vi "Process.vi"(8 "error in":errorcluster, 11 "SMO.DynamicLauncher":refnum<class "SMO.DynamicLauncher.lvclass">) -> (0 "error out":errorcluster, 3 "SMO.DynamicLauncher out":refnum<class "SMO.DynamicLauncher.lvclass">)   [LabVIEW 2021, in "SMO.DynamicLauncher.lvclass"]
doc: "---------------------------------------------------------------\nJKI State Machine Objects™\nhttp://jki.net/state-machine-objects/\nCopyright (C) 2005-2015, JKI <info@jki.net>\nALL RIGHTS RESERVED"
uses:
  SMO.DynamicLauncher.lvclass
  SMO.DynamicLauncher.lvclass/SMO.DynamicLauncher.ctl
  src/SMO/SMO.lvclass
  C:/Repositories/SMO/src/SMO/SMO.lvclass
  C:/Repositories/SMO/tests/_test-support-SMOs/SMO.DynamicLauncher/SMO.DynamicLauncher.lvclass
  src/SMO/Typedefs/SMOState --Enum.ctl
panel:
  # "For instructions on how to use the JKI State Machine Objects, examples and video tutorials, visit:\nhttp://jki.net/state-machine-objects/\n\nJKI State Machine Objects™\nhttp://jki.net/state-machine-objects/\nCopyright (C) 2005-2015, JKI <info@jki.net>\nALL RIGHTS RESERVED"
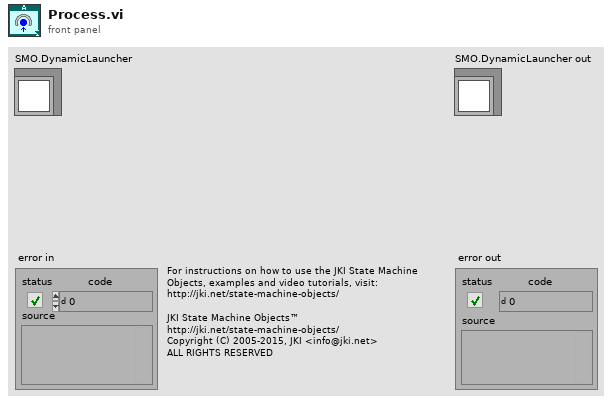
[diagram p1: front panel]
types:
  T1 = enum32{"invalid app kind", "Development System", "Run Time System", "Student Edition", "Embedded LabVIEW", "Evaluation", "Custom"}
  T2 = enum32{"Invalid", "Standard", "Closed", "Hidden", "Minimized", "Maximized"}
  T3 = typedef "smo.lvlib/SMO.lvclass/SMOState --Enum.ctl" = enum16{"unknown", "Created", "Started", "Stopped"}
  T4 = cluster{"Core":cluster{"Current VI Reference":refnum<vi>, "Close Panel on Exit?":bool, "error":errorcluster}, "SelfRef":refnum<class "SMO.DynamicLauncher.lvclass">}
  T5 = cluster{"Current VI Reference":refnum<vi>, "Close Panel on Exit?":bool, "error":errorcluster}
  T6 = typedef "smo.lvlib/SMO.lvclass/Protected Events.ctl" = cluster{"StopProcesses":refnum<user-event>, "AbortProcesses":refnum<user-event>, "Config Changed":refnum<user-event>, "Dependency":refnum<user-event>}
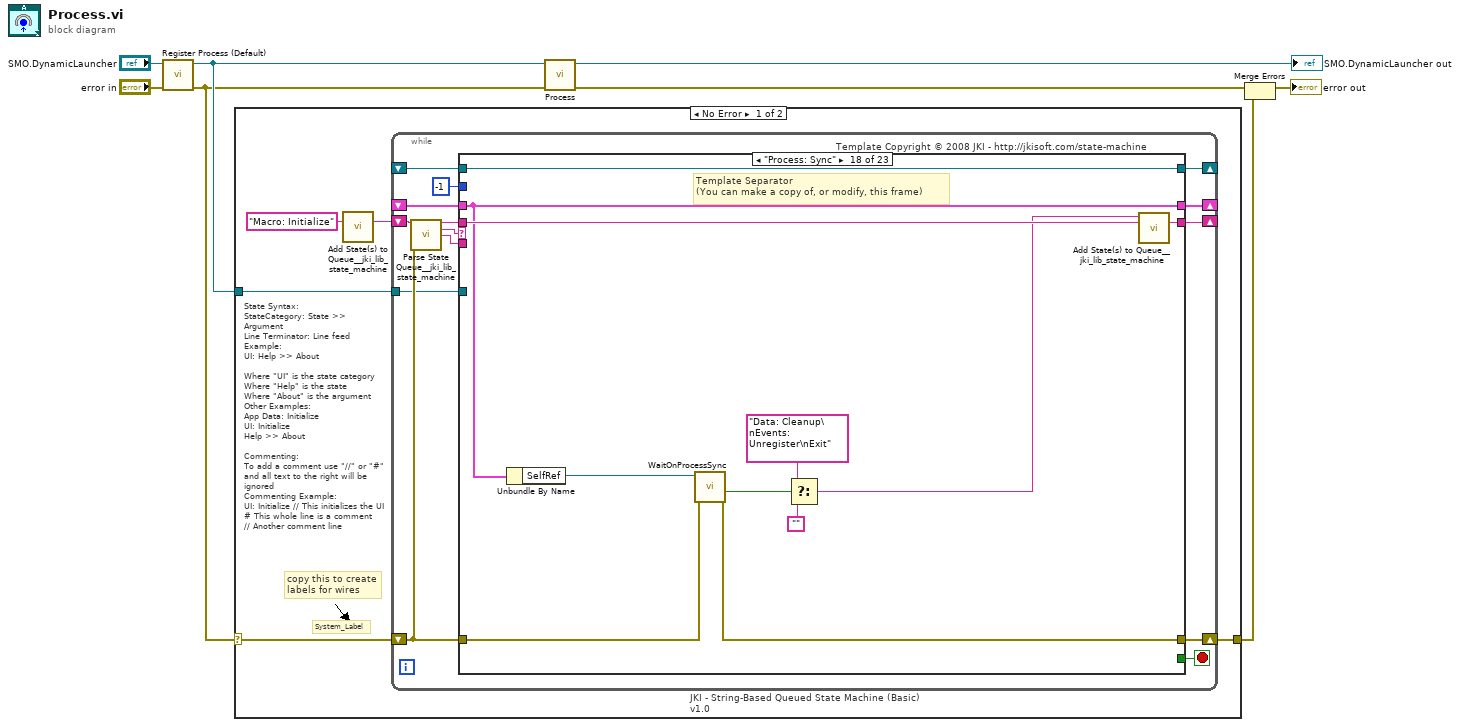
[diagram p0: block diagram]
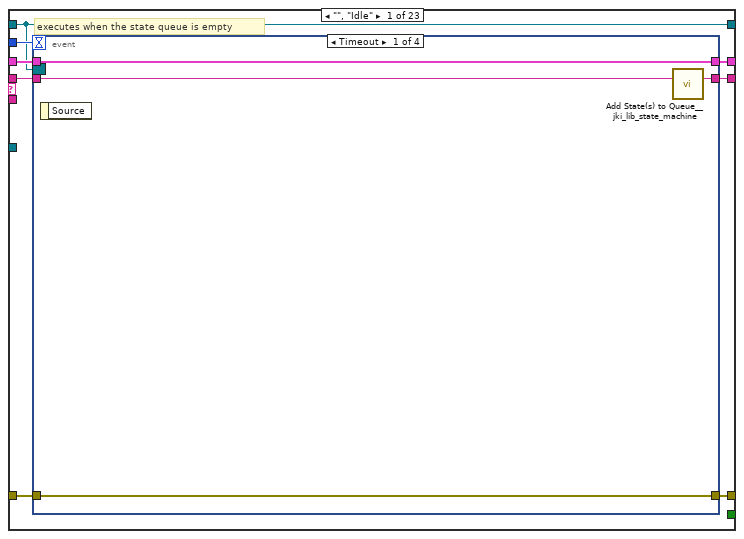
[diagram p2: hidden frame]
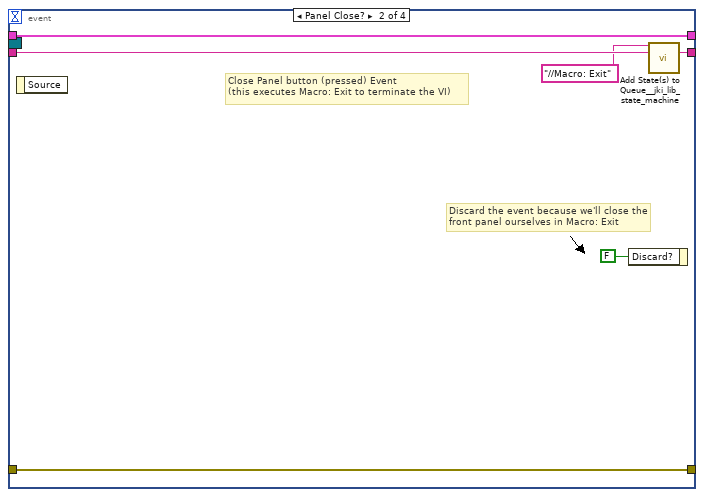
[diagram p3: hidden frame]
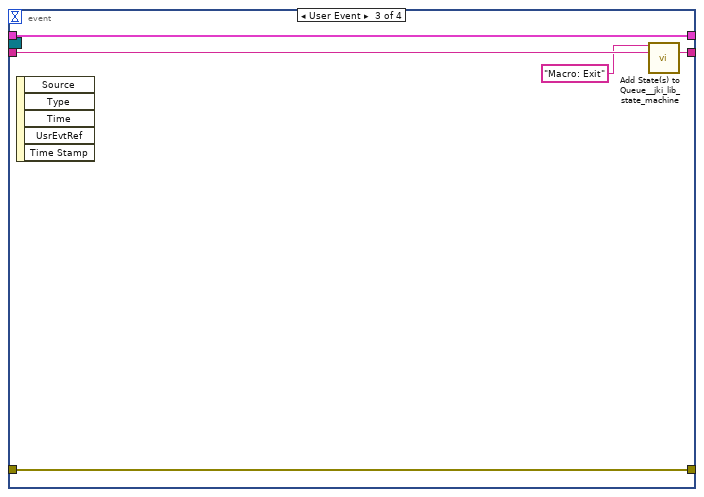
[diagram p4: hidden frame]
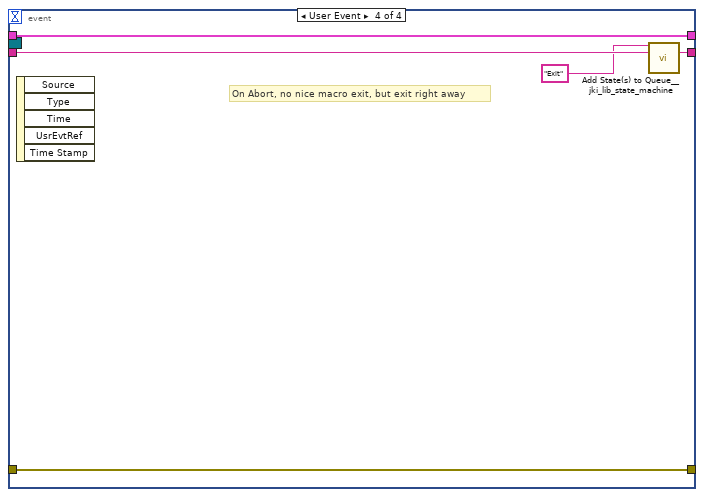
[diagram p5: hidden frame]
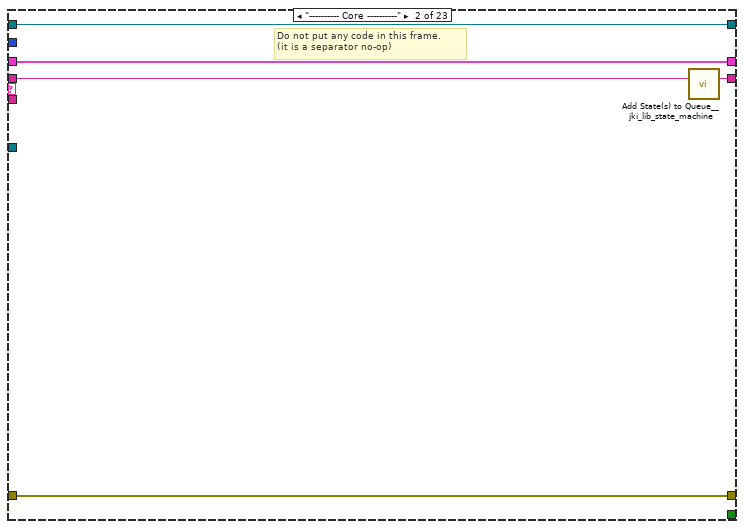
[diagram p6: hidden frame]
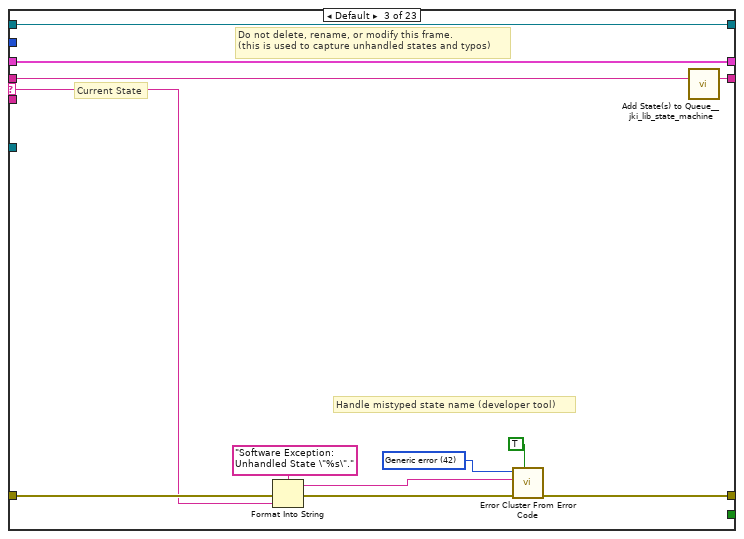
[diagram p7: hidden frame]
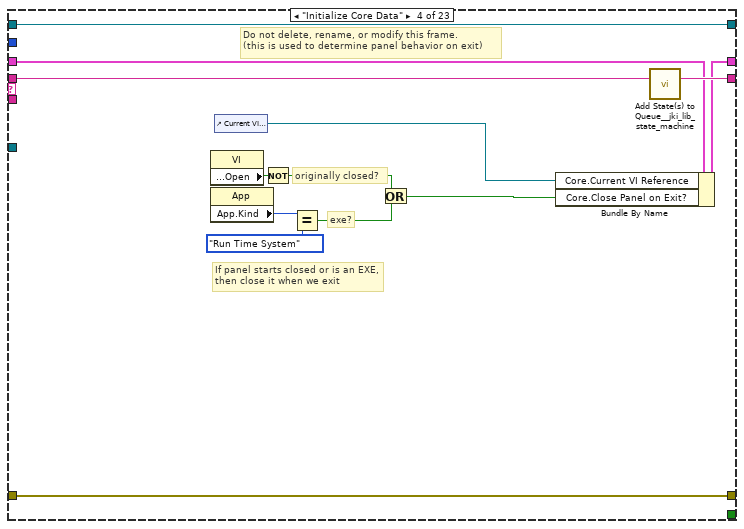
[diagram p8: hidden frame]
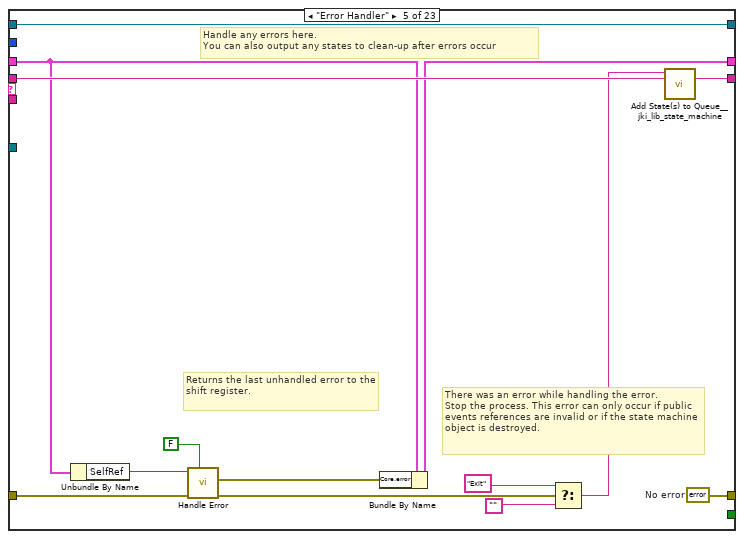
[diagram p9: hidden frame]
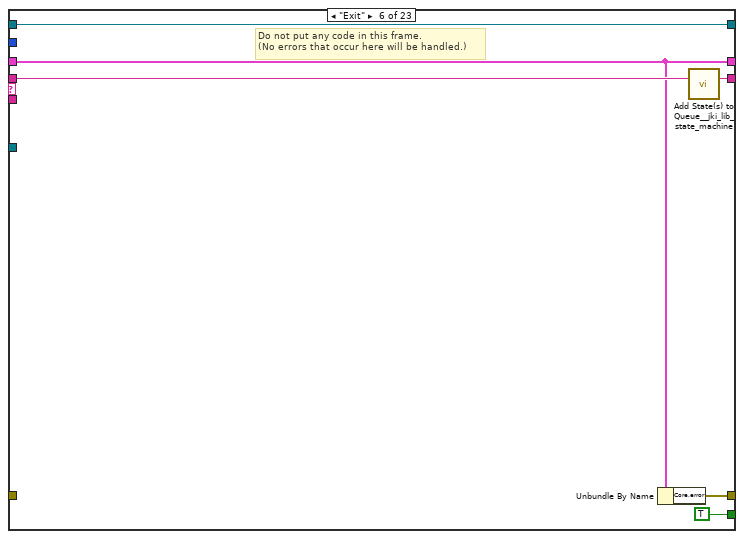
[diagram p10: hidden frame]
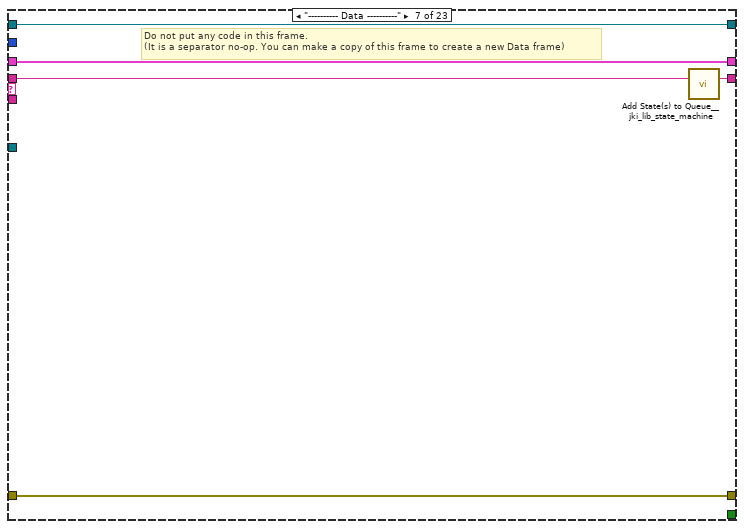
[diagram p11: hidden frame]
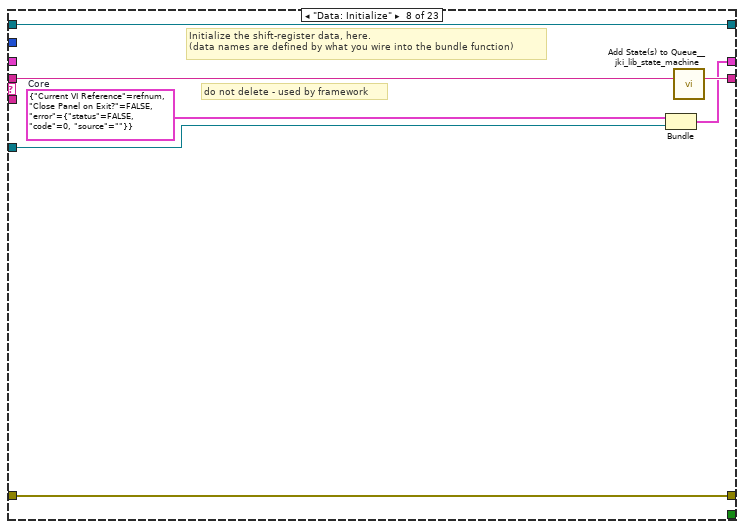
[diagram p12: hidden frame]
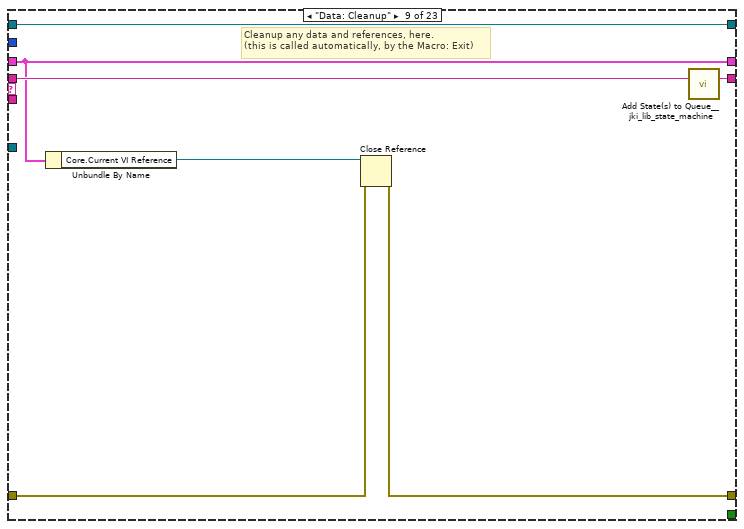
[diagram p13: hidden frame]
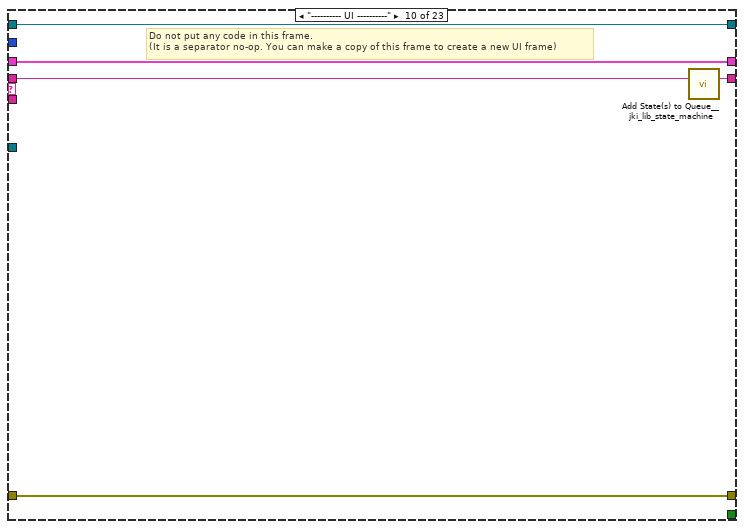
[diagram p14: hidden frame]
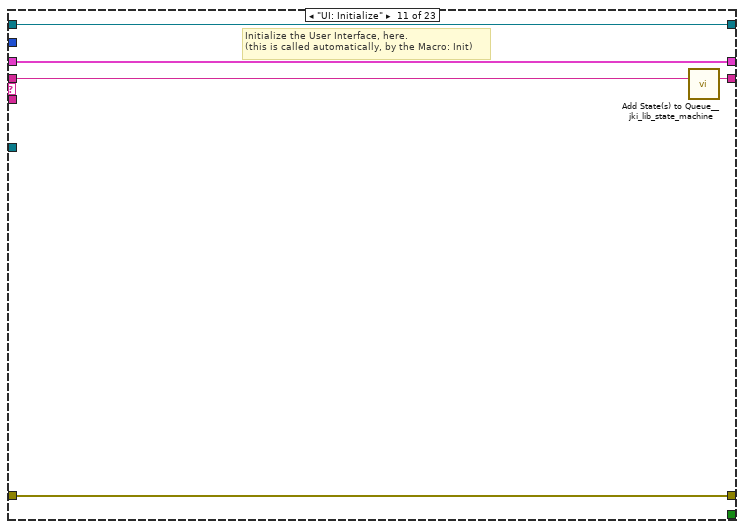
[diagram p15: hidden frame]
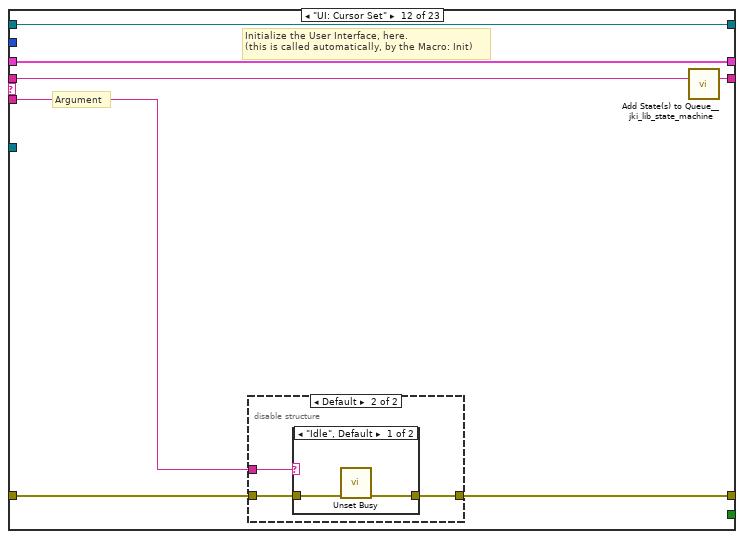
[diagram p16: hidden frame]
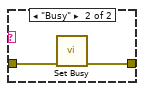
[diagram p18: hidden frame]
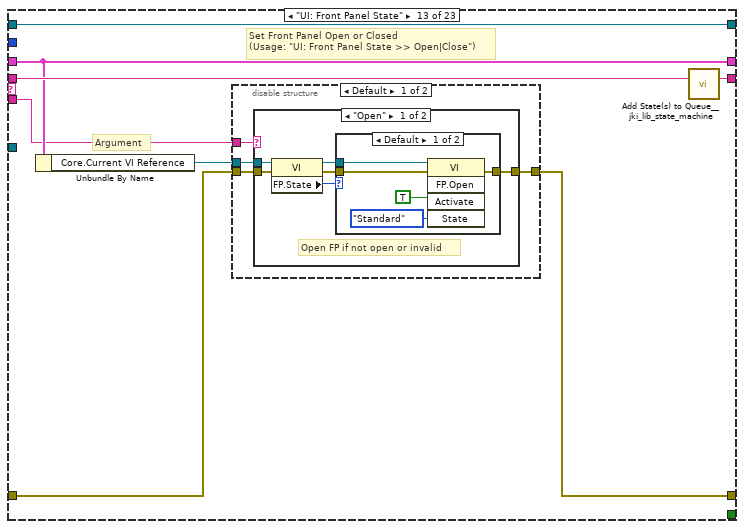
[diagram p19: hidden frame]
diagram:
  n1 = call "Register Process (Default).vi"("error in (no error)"="error in", "SMO"="SMO.DynamicLauncher") -> ("error out"=w1:errorcluster, "SelfRef"=w3:refnum<class "SMO.DynamicLauncher.lvclass">)  [unwired: 8 in]
  n2 = case shown="No Error" w1 {
    selector: w1 -> [w10 w278]
    tunnel: w3 -> [w11 _]
    tunnel: [w9 w278] -> w5
    frame No Error {
      # "State Syntax:\nStateCategory: State >> Argument\nLine Terminator: Line feed\nExample:\nUI: Help >> About\n\nWhere \"UI\" is the state category\nWhere \"Help\" is the state\nWhere \"About\" is the argument\nOther Examples:\nApp Data: Initialize\nUI: Initialize\nHelp >> About\n\nCommenting:\nTo add a comment use \"//\" or \"#\" and all text to the right will be ignored\nCommenting Example:\nUI: Initialize // This initializes the UI\n# This whole line is a comment\n// Another comment line"
      # "copy this to create labels for wires"
      # "System_Label"
      n3 = call <vilib>:"Add State(s) to Queue__jki_lib_state_machine.vi"("State(s) in (\"\")"="Macro: Initialize") -> ("States Out"=w13:string)  [unwired: 14 in]
      n4 = while "JKI - String-Based Queued State Machine (Basic) v1.0" {
        shift-right: [w20] -> _
        shift-left: _ -> [w19]
        shift-right: [w23] -> w9
        shift-left: w10 -> [w17]
        shift-right: [w22] -> _
        shift-left: w13 -> [w24]
        tunnel: w11 -> [w16]
        shift-right: [w15] -> _
        shift-left: _ -> [w14]
        stop <- w21 stop-if-true
        # "Template Copyright © 2008 JKI - http://jkisoft.com/state-machine"
        n5 = call <vilib>:"Parse State Queue__jki_lib_state_machine.vi"("State Queue"=w24, "Error In (no error)"=w17) -> ("Remaining States"=w26:string, "Current State"=w27:string, "Arguments"=w25:string)  [unwired: 11 in]
        n6 = case shown="\"Process: Sync\"" w27 {
          selector: w27 -> [_ _ w62 _ _ _ _ _ _ _ _ _ _ _ _ _ _ _ _ _ _ _ _]
          tunnel: w26 -> [w35 w60 w66 w85 w99 w105 w110 w117 w124 w129 w134 w141 w157 w189 w198 w212 w217 w228 w233 w243 w249 w254 w266]
          tunnel: w25 -> [_ _ _ _ _ _ _ _ _ _ _ w135 w150 _ _ _ _ _ _ _ _ _ _]
          tunnel: w19 -> [w33 w57 w64 w76 w90 w101 w107 _ w119 w126 w132 w139 w155 w186 w194 w203 w214 w225 w230 w241 w247 w252 w263]
          tunnel: [w32 w58 w68 w82 w87 w100 w108 w111 w120 w127 w131 w136 w151 w187 w196 w210 w215 w219 w231 w234 w245 w250 w259] -> w23
          tunnel: w17 -> [w31 w58 w67 w82 w91 _ w108 w111 w121 w127 w131 w137 w152 w187 w196 w210 w215 w220 w231 w235 w245 w250 w260]
          tunnel: [w34 w59 w65 w84 w98 w104 w109 w116 w123 w128 w133 w140 w156 w188 w197 w211 w216 w227 w232 w242 w248 w253 w265] -> w22
          tunnel: [_ _ _ _ _ TRUE _ _ _ _ _ _ _ _ _ _ _ _ _ _ _ _ _] -> w21
          tunnel: [w30 w57 w64 w83 w89 w101 w107 w115 w119 w126 w132 w139 w155 w186 w194 w203 w214 w225 w230 w241 w247 w252 w263] -> w20
          tunnel: -1 -> [w29 _ _ _ _ _ _ _ _ _ _ _ _ _ _ _ _ _ _ _ _ _ _]
          tunnel: w16 -> [_ _ _ _ _ _ _ w112 _ _ _ _ _ _ _ _ _ _ _ _ _ _ _]
          tunnel: [w28 w56 w61 w73 w97 w102 w106 w114 w118 w125 w130 w138 w154 w185 w195 w204 w213 w226 w229 w238 w246 w251 w264] -> w15
          tunnel: w14 -> [w28 w56 w61 w73 w97 w102 w106 w114 w118 w125 w130 w138 w154 w185 w195 w204 w213 w226 w229 _ w246 w251 w264]
          frame "", "Idle" {
            # "executes when the state queue is empty"
            n7 = event shown="[0] Timeout" {
              selector: w28 -> [_ _ _ _]
              dyn-events: _ -> [_ _ _ _]
              timeout: w29 -> [_ _ _ _]
              tunnel: w35 -> [w39 w45 w50 w55]
              tunnel: [w38 w44 w49 w54] -> w34
              tunnel: w33 -> [w36 w42 w47 w52]
              tunnel: [w37 w43 w48 w53] -> w32
              tunnel: w31 -> [w37 w43 w48 w53]
              tunnel: [w36 w42 w47 w52] -> w30
              event Timeout {
                n8 = event-data() -> ()  [unwired: 1 in, 1 out]
                n9 = call <vilib>:"Add State(s) to Queue__jki_lib_state_machine.vi"("State(s) in (\"\")"=w39) -> ("States Out"=w38:string)  [unwired: 14 in]
              }
              event Panel Close? {
                # "Discard the event because we'll close the front panel ourselves in Macro: Exit"
                # "Close Panel button (pressed) Event\n(this executes Macro: Exit to terminate the VI)"
                n10 = event-data() -> ()  [unwired: 1 in, 1 out]
                n11 = event-data("Discard?"=FALSE) -> ()  [unwired: 1 in, 1 out]
                n12 = call <vilib>:"Add State(s) to Queue__jki_lib_state_machine.vi"("State(s) in Front (\"\")"="//Macro: Exit", "State(s) in (\"\")"=w45) -> ("States Out"=w44:string)  [unwired: 13 in]
              }
              event User Event {
                n13 = event-data() -> ()  [unwired: 1 in, 5 out]
                n14 = call <vilib>:"Add State(s) to Queue__jki_lib_state_machine.vi"("State(s) in Front (\"\")"="Macro: Exit", "State(s) in (\"\")"=w50) -> ("States Out"=w49:string)  [unwired: 13 in]
              }
              event User Event {
                # "On Abort, no nice macro exit, but exit right away"
                n15 = event-data() -> ()  [unwired: 1 in, 5 out]
                n16 = call <vilib>:"Add State(s) to Queue__jki_lib_state_machine.vi"("State(s) in Front (\"\")"="Exit", "State(s) in (\"\")"=w55) -> ("States Out"=w54:string)  [unwired: 13 in]
              }
            }
          }
          frame "---------- Core ----------" {
            # "Do not put any code in this frame.\n(it is a separator no-op)"
            n17 = call <vilib>:"Add State(s) to Queue__jki_lib_state_machine.vi"("State(s) in (\"\")"=w60) -> ("States Out"=w59:string)  [unwired: 14 in]
          }
          frame Default {
            w71 = 42 items=["No error", "Argument error", "Memory is full", "Out of zone", "End of file", "File already open", "Generic file I/O error", "File not found", "File permission error", "Disk is full", "Duplicate path", "Too many files open", "System feature not enabled", "Resource file not found", "Cannot add resource", "Resource not found", "Image not found", "Image memory error", "Pen does not exist", "Config type invalid", "Config token not found", "Config parse error", "Config memory error", "Bad external code format", "Bad external code offset", "External code not present", "Null window", "Destroy window error", "Null menu", "Print aborted", "Bad print record", "Print driver error", "Windows error during printing", "Memory error during printing", "Print dialog error", "Generic print error", "Invalid device refnum", "Device not found", "Device parameter error", "Device unit error", "Cannot open device", "Device call aborted", "Generic error", "Cancelled by user", "Object ID too low", "Object ID too high", "Object not in heap", "Unknown heap", "Unknown object (invalid DefProc)", "Unknown object (DefProc not in table)", "Message out of range", "Invalid (null) method", "Unknown message", "Manager call not supported", "Bad address", "Network operation in progress", "Network operation timed out", "Connection is busy", "Network attribute not supported", "Network error", "Address in use", "System out of memory", "Connection aborted", "Connection refused", "Not connected", "Already connected", "Connection closed", "Initialization error (interapplication manager)", "Bad occurrence", "Wait on unbound occurrence handler", "Occurrence queue overflow", "Datalog type conflict", "Unused", "Unrecognized type (interapplication manager)", "Memory corrupt", "Failed to make temporary DLL", "Old CIN version", "Drag socket not found", "Failed to load drop-object", "Failed to register OLE object", "Failed to release OLE object", "Format specifier type mismatch", "Unknown format specifier", "Too few format specifiers", "Too many format specifiers", "Scan failed", "Newer CIN version", "Error converting to variant", "Runtime menu error", "Password tampered", "Variant attribute not found", "Incompatible variant data type", "Event data is not available", "Event Store is not present", "Occurrence is not found", "Event Queue is not created", "Event info is not available", "Refnum passed is NULL", "Error retrieving Class GUID", "Error retrieving CoClass GUID", "Error retrieving TypeLib GUID.", "Bad built application magic bytes.", "Specific driver is different from the specific driver associated with the Logical Name.", "There is no session opened to the class driver.", "Max Error", "MAX - Error with config objects", "MAX - Error loading configuration", "MAX - Group not supported"]
            # "Current State"
            # "Do not delete, rename, or modify this frame.\n(this is used to capture unhandled states and typos)"
            # "Handle mistyped state name (developer tool)"
            n18 = Format Into String(format string="Software Exception: Unhandled State \"%s\"." ("message"), error in=w67, w62) -> (resulting string=w70:string, error out=w69:errorcluster)  [unwired: 1 in]
            n19 = call <vilib>:"Error Cluster From Error Code.vi"("show call chain? (False)"=TRUE, "error in (no error)"=w69, "error message (\"\")"=w70, "error code (0)"=w71) -> ("error out"=w68:errorcluster)  [unwired: 5 in]
            n20 = call <vilib>:"Add State(s) to Queue__jki_lib_state_machine.vi"("State(s) in (\"\")"=w66) -> ("States Out"=w65:string)  [unwired: 14 in]
          }
          frame "Initialize Core Data" {
            # "Do not delete, rename, or modify this frame.\n(this is used to determine panel behavior on exit)"
            # "originally closed?"
            # "exe?"
            # "If panel starts closed or is an EXE, then close it when we exit"
            n21 = property class="VI"() -> ("Front Panel.Open"=w81:bool)  [unwired: 2 in, 2 out]
            n22 = property class="App"() -> ("App.Kind"=w80:T1)  [unwired: 2 in, 2 out]
            n23 = control-ref of="Current VI Reference"() -> (w74:refnum<vi>)
            n24 = Not(x=w81) -> (.not. x?=w78:bool)
            n25 = Equal?(x=w80, y=T1."Run Time System" ("Application:Kind")) -> (x = y?=w77:bool)
            n26 = Or(x=w78, y=w77) -> (x .or. y?=w75:bool)
            n27 = Bundle By Name(cluster=w76, "Core.Current VI Reference"=w74, "Core.Close Panel on Exit?"=w75) -> (w83:T4)
            n28 = call <vilib>:"Add State(s) to Queue__jki_lib_state_machine.vi"("State(s) in (\"\")"=w85) -> ("States Out"=w84:string)  [unwired: 14 in]
          }
          frame "Error Handler" {
            w87 = errorcluster {"status"=FALSE, "code"=0, "source"=""}  # No error
            # "Returns the last unhandled error to the shift register."
            # "There was an error while handling the error.\nStop the process. This error can only occur if public events references are invalid or if the state machine object is destroyed."
            # "Handle any errors here.\nYou can also output any states to clean-up after errors occur"
            n29 = Unbundle By Name(w90) -> ("SelfRef"=w92:refnum<class "SMO.DynamicLauncher.lvclass">)
            n30 = call-dynamic "Handle Error.vi"("Stop on Unhandled Error (T)"=FALSE, "error in"=w91, "SMO"=w92) -> ("handling error"=w94:errorcluster, "Unhandled error"=w93:errorcluster)  [unwired: 6 in, 1 out]
            n31 = Bundle By Name(cluster=w90, "Core.error"=w93) -> (w89:T4)
            n32 = Select(t="Exit", s=w94, f="") -> (s? t:f=w88:string)
            n33 = call <vilib>:"Add State(s) to Queue__jki_lib_state_machine.vi"("State(s) in Front (\"\")"=w88, "State(s) in (\"\")"=w99) -> ("States Out"=w98:string)  [unwired: 13 in]
          }
          frame "Exit" {
            # "Do not put any code in this frame.\n(No errors that occur here will be handled.)"
            n34 = Unbundle By Name(w101) -> ("Core.error"=w100:errorcluster)
            n35 = call <vilib>:"Add State(s) to Queue__jki_lib_state_machine.vi"("State(s) in (\"\")"=w105) -> ("States Out"=w104:string)  [unwired: 14 in]
          }
          frame "---------- Data ----------" {
            # "Do not put any code in this frame.\n(It is a separator no-op. You can make a copy of this frame to create a new Data frame)"
            n36 = call <vilib>:"Add State(s) to Queue__jki_lib_state_machine.vi"("State(s) in (\"\")"=w110) -> ("States Out"=w109:string)  [unwired: 14 in]
          }
          frame "Data: Initialize" {
            w113 = T5 {"Current VI Reference"=refnum, "Close Panel on Exit?"=FALSE, "error"={"status"=FALSE, "code"=0, "source"=""}}  # Core
            # "do not delete - used by framework"
            # "Initialize the shift-register data, here.\n(data names are defined by what you wire into the bundle function)"
            n37 = Bundle("Core"=w113, "SelfRef"=w112) -> (w115:T4)  [unwired: 1 in]
            n38 = call <vilib>:"Add State(s) to Queue__jki_lib_state_machine.vi"("State(s) in (\"\")"=w117) -> ("States Out"=w116:string)  [unwired: 14 in]
          }
          frame "Data: Cleanup" {
            # "Cleanup any data and references, here.\n(this is called automatically, by the Macro: Exit)"
            n39 = Unbundle By Name(w119) -> ("Core.Current VI Reference"=w122:refnum<vi>)
            n40 = Close Reference(reference=w122, error in (no error)=w121) -> (error out=w120:errorcluster)
            n41 = call <vilib>:"Add State(s) to Queue__jki_lib_state_machine.vi"("State(s) in (\"\")"=w124) -> ("States Out"=w123:string)  [unwired: 14 in]
          }
          frame "---------- UI ----------" {
            # "Do not put any code in this frame.\n(It is a separator no-op. You can make a copy of this frame to create a new UI frame)"
            n42 = call <vilib>:"Add State(s) to Queue__jki_lib_state_machine.vi"("State(s) in (\"\")"=w129) -> ("States Out"=w128:string)  [unwired: 14 in]
          }
          frame "UI: Initialize" {
            # "Initialize the User Interface, here.\n(this is called automatically, by the Macro: Init)"
            n43 = call <vilib>:"Add State(s) to Queue__jki_lib_state_machine.vi"("State(s) in (\"\")"=w134) -> ("States Out"=w133:string)  [unwired: 14 in]
          }
          frame "UI: Cursor Set" {
            # "Argument"
            # "Initialize the User Interface, here.\n(this is called automatically, by the Macro: Init)"
            n44 = disable-structure shown="Default" {
              disable-tunnel: w137 -> [w142 w145]
              disable-tunnel: [w142 w144] -> w136
              disable-tunnel: w135 -> [_ w143]
              frame condition #0 {
              }
              frame condition #1 (active) {
                n45 = case shown="\"Idle\", Default" w143 {
                  tunnel: w145 -> [w147 w149]
                  tunnel: [w146 w148] -> w144
                  frame "Idle", Default {
                    n46 = call <vilib>:"Unset Busy.vi"("error in (no error)"=w147) -> ("error out"=w146:errorcluster)  [unwired: 10 in]
                  }
                  frame "Busy" {
                    n47 = call <vilib>:"Set Busy.vi"("error in (no error)"=w149) -> ("error out"=w148:errorcluster)  [unwired: 9 in, 1 out]
                  }
                }
              }
            }
            n48 = call <vilib>:"Add State(s) to Queue__jki_lib_state_machine.vi"("State(s) in (\"\")"=w141) -> ("States Out"=w140:string)  [unwired: 14 in]
          }
          frame "UI: Front Panel State" {
            # "Argument"
            # "Set Front Panel Open or Closed\n(Usage: \"UI: Front Panel State >> Open|Close\")"
            n49 = Unbundle By Name(w155) -> ("Core.Current VI Reference"=w153:refnum<vi>)
            n50 = disable-structure shown="Default" {
              disable-tunnel: w152 -> [w161 w184]
              disable-tunnel: [w160 w184] -> w151
              disable-tunnel: w153 -> [w159 _]
              disable-tunnel: w150 -> [w158 _]
              frame condition #0 (active) {
                n51 = case shown="\"Open\"" w158 {
                  tunnel: w161 -> [w165 w178]
                  tunnel: [w167 w179] -> w160
                  tunnel: w159 -> [w166 w176]
                  frame "Open" {
                    # "Open FP if not open or invalid"
                    n52 = property class="VI"(reference=w166, error in=w165) -> (reference out=w163:refnum<vi>, error out=w164:errorcluster, "FP.State"=w162:T2)
                    n53 = case shown="Default" w162 {
                      tunnel: [w170 w173] -> w167
                      tunnel: w164 -> [w169 w173]
                      tunnel: w163 -> [w168 _]
                      frame Default {
                        n54 = invoke class="VI" method="FP.Open"(reference=w168, error in=w169, "Activate"=TRUE, "State"=T2."Standard") -> (error out=w170:errorcluster)  [unwired: 1 in, 4 out]
                      }
                      frame "Invalid", "Standard" {
                      }
                    }
                  }
                  frame "Close", Default {
                    # "Close FP is not Closed or Invalid"
                    n55 = property class="VI"(reference=w176, error in=w178) -> (reference out=w175:refnum<vi>, error out=w177:errorcluster, "FP.State"=w174:T2)
                    n56 = case shown="Default" w174 {
                      tunnel: [w180 w183] -> w179
                      tunnel: w177 -> [w180 w182]
                      tunnel: w175 -> [_ w181]
                      frame "Invalid", "Closed" {
                      }
                      frame Default {
                        n57 = invoke class="VI" method="FP.Close"(reference=w181, error in=w182) -> (error out=w183:errorcluster)  [unwired: 1 in, 2 out]
                      }
                    }
                  }
                }
              }
              frame condition #1 {
              }
            }
            n58 = call <vilib>:"Add State(s) to Queue__jki_lib_state_machine.vi"("State(s) in (\"\")"=w157) -> ("States Out"=w156:string)  [unwired: 14 in]
          }
          frame "---------- Macro ----------" {
            # "Do not put any code in this frame.\n(It is a separator no-op. You can make a copy of this frame to create a new Macro frame)"
            n59 = call <vilib>:"Add State(s) to Queue__jki_lib_state_machine.vi"("State(s) in (\"\")"=w189) -> ("States Out"=w188:string)  [unwired: 14 in]
          }
          frame "Macro: Initialize" {
            # "Initialization Macro\n(This is called once, when the VI starts)"
            n60 = call <vilib>:"Add State(s) to Queue__jki_lib_state_machine.vi"("State(s) in Front (\"\")"="Data: Initialize\nInitialize Core Data\nEvents: Register", "State(s) in (\"\")"="Process: Sync", "State(s) at Back (\"\")"="UI: Initialize\nAction: Launch Dynamically") -> ("States Out"=w191:string)  [unwired: 12 in]
            n61 = call <vilib>:"Add State(s) to Queue__jki_lib_state_machine.vi"("State(s) in Front (\"\")"=w191, "State(s) in (\"\")"=w198) -> ("States Out"=w197:string)  [unwired: 13 in]
          }
          frame "Macro: Exit" {
            # "Exit Macro\n(This is called once, when the VI exits)"
            n62 = Unbundle By Name(w203) -> ("Core.Close Panel on Exit?"=w209:bool)
            n63 = Select(t="//UI: Front Panel State >> Close", s=w209, f="") -> (s? t:f=w206:string)
            n64 = call <vilib>:"Add State(s) to Queue__jki_lib_state_machine.vi"("State(s) in Front (\"\")"="Data: Cleanup\nEvents: Unregister", "State(s) in (\"\")"="Process: Sync", "State(s) at Back (\"\")"="Exit") -> ("States Out"=w200:string)  [unwired: 12 in]
            n65 = call <vilib>:"Add State(s) to Queue__jki_lib_state_machine.vi"("State(s) in (\"\")"=w206, "State(s) at Back (\"\")"=w200) -> ("States Out"=w205:string)  [unwired: 13 in]
            n66 = call <vilib>:"Add State(s) to Queue__jki_lib_state_machine.vi"("State(s) in Front (\"\")"=w205, "State(s) in (\"\")"=w212) -> ("States Out"=w211:string)  [unwired: 13 in]
          }
          frame "---------- Process ----------" {
            # "Template Separator\n(You can make a copy of, or modify, this frame)"
            n67 = call <vilib>:"Add State(s) to Queue__jki_lib_state_machine.vi"("State(s) in (\"\")"=w217) -> ("States Out"=w216:string)  [unwired: 14 in]
          }
          frame "Process: Sync" {
            # "Template Separator\n(You can make a copy of, or modify, this frame)"
            n68 = Unbundle By Name(w225) -> ("SelfRef"=w221:refnum<class "SMO.DynamicLauncher.lvclass">)
            n69 = call "WaitOnProcessSync.vi"("error in (no error)"=w220, "SMO"=w221) -> ("error out"=w219:errorcluster, "Don't run?"=w224:bool)  [unwired: 7 in, 1 out]
            n70 = Select(t="Data: Cleanup\nEvents: Unregister\nExit", s=w224, f="") -> (s? t:f=w218:string)
            n71 = call <vilib>:"Add State(s) to Queue__jki_lib_state_machine.vi"("State(s) in Front (\"\")"=w218, "State(s) in (\"\")"=w228) -> ("States Out"=w227:string)  [unwired: 13 in]
          }
          frame "---------- Events ----------" {
            # "Template Separator\n(You can make a copy of, or modify, this frame)"
            n72 = call <vilib>:"Add State(s) to Queue__jki_lib_state_machine.vi"("State(s) in (\"\")"=w233) -> ("States Out"=w232:string)  [unwired: 14 in]
          }
          frame "Events: Register" {
            # "Self Public Events"
            # "Base Class Protected Events"
            # "Your code here.\n(You can make a copy of, or modify, this frame)"
            n73 = Unbundle By Name(w241) -> ("SelfRef"=w240:refnum<class "SMO.DynamicLauncher.lvclass">)
            n74 = call "GetProtectedEvents.vi"("SMO"=w240) -> ("error out"=w236:errorcluster, "SMO Protected Events"=w239:T6)  [unwired: 8 in, 1 out]
            n75 = register-events(w239) -> (reference out=w238:refnum<event-registration>, error out=w237:errorcluster)  [unwired: 2 in]
            n76 = Merge Errors(w235, w237, w236) -> (w234:errorcluster)
            n77 = call <vilib>:"Add State(s) to Queue__jki_lib_state_machine.vi"("State(s) in (\"\")"=w243) -> ("States Out"=w242:string)  [unwired: 14 in]
          }
          frame "Events: Unregister" {
            # "Your code here.\n(You can make a copy of, or modify, this frame)"
            n78 = Unregister For Events(event registration refnum=w246, error in=w245) -> (error out=w244:errorcluster)
            n79 = call <vilib>:"Clear Errors.vi"("error in (no error)"=w244) -> ()  [unwired: 5 in, 2 out]
            n80 = call <vilib>:"Add State(s) to Queue__jki_lib_state_machine.vi"("State(s) in (\"\")"=w249) -> ("States Out"=w248:string)  [unwired: 14 in]
          }
          frame "---------- Action ----------" {
            n81 = call <vilib>:"Add State(s) to Queue__jki_lib_state_machine.vi"("State(s) in (\"\")"=w254) -> ("States Out"=w253:string)  [unwired: 14 in]
          }
          frame "Action: Launch Dynamically" {
            n82 = Unbundle By Name(w263) -> ("SelfRef"=w258:refnum<class "SMO.DynamicLauncher.lvclass">)
            n83 = call "Read WaitStarted.vi"("SMO.DynamicLauncher in"=w258) -> ("WaitStarted"=w255:bool, "SMO.DynamicLauncher out"=w257:refnum<class "SMO.DynamicLauncher.lvclass">)  [unwired: 9 in]
            n84 = case shown="True" w255 {
              tunnel: w257 -> [w267 w271]
              tunnel: [w267 w270] -> w256
              frame False {
              }
              frame True {
                n85 = call "WaitForState.vi"("timeout in ms (-1)"=2000, "State (unknown: any state)"=SMOState_--Enum."Started" ("SMO State"), "SMO in"=w271) -> ("SMO out"=w270:refnum<class "SMO.DynamicLauncher.lvclass">)  [unwired: 6 in, 2 out]
              }
            }
            n86 = for {
              N: 10 -> [_]
              tunnel: w256 -> [w277]
              tunnel: [w273] -> w261 mode=indexing
              i -> [w276]
              n87 = Format Into String(format string="temp_%d", w276) -> (resulting string=w274:string)  [unwired: 2 in, 1 out]
              n88 = call "LaunchDependency.vi"("Dependency Name"=w274, "Dependency Type"=refnum<class "SMO.lvclass"> refnum ("smo.lvlib:SMO.lvclass"), "SMO in"=w277) -> ("error out"=w273:errorcluster)  [unwired: 5 in, 3 out]
            }
            n89 = Merge Errors(w260, w261) -> (w259:errorcluster)
            n90 = call <vilib>:"Add State(s) to Queue__jki_lib_state_machine.vi"("State(s) in (\"\")"=w266) -> ("States Out"=w265:string)  [unwired: 14 in]
          }
        }
      }
    }
    frame Error {
    }
  }
  n91 = call-parent "Process.vi"("error in"=w1, "SMO"=w3) -> ("error out"=w6:errorcluster, "SMO out"=→"SMO.DynamicLauncher out":refnum<class "SMO.DynamicLauncher.lvclass">)  [unwired: 8 in]
  n92 = Merge Errors(w6, w5) -> (→"error out":errorcluster)
